vi "0816039.vi"() -> ()   [LabVIEW 2021]
panel:
  out "M2":string
  out "M1":string
  out "elapsed\ntime":u32
  out "current time":timestamp format="%<%X %x>T"
  in  "stop":bool
  out "Display":string
  in  "Calculator":T1
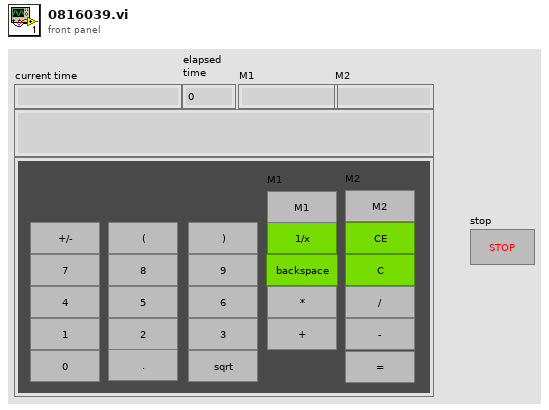
[diagram p1: front panel]
types:
  T1 = cluster{"1":bool, "2":bool, "3":bool, "4":bool, "5":bool, "6":bool, "7":bool, "8":bool, "9":bool, "+":bool, "-":bool, "*":bool, "/":bool, "C":bool, "=":bool, "0":bool, ".":bool, "(":bool, ")":bool, "backspace":bool, "1/x":bool, "CE":bool, "sqrt":bool, "+/-":bool, "M1":bool, "M2":bool}
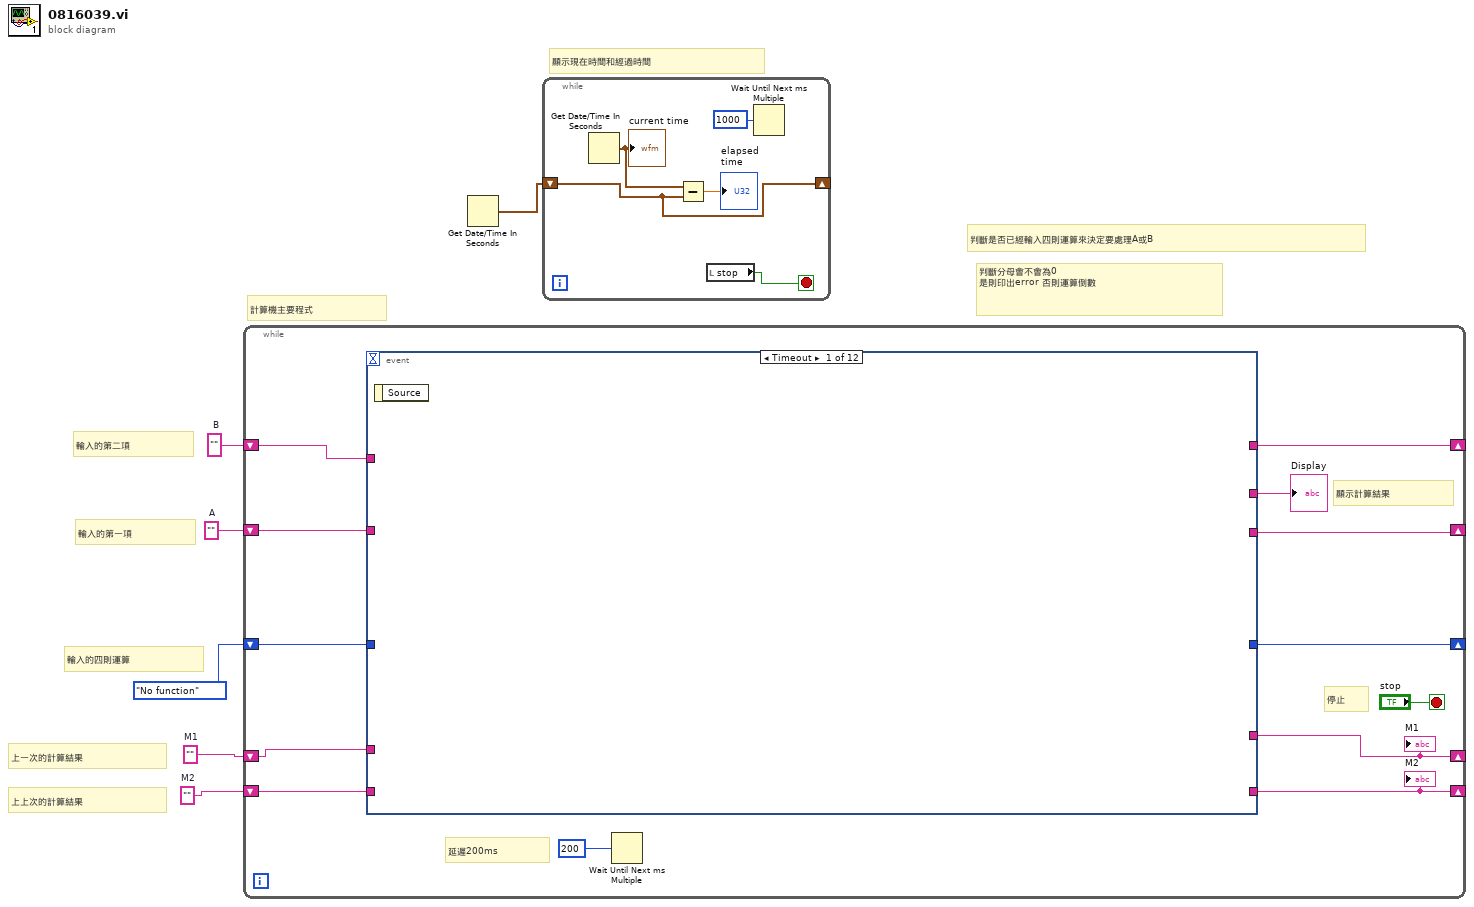
[diagram p0: block diagram]
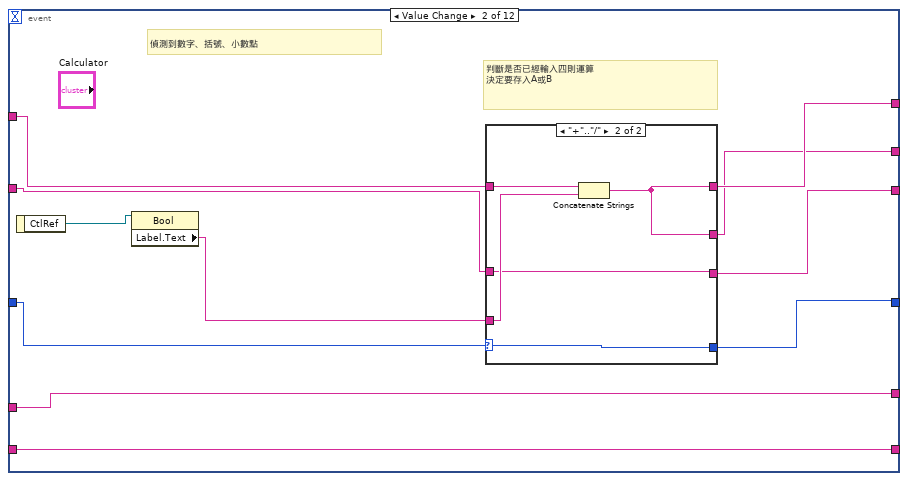
[diagram p2: hidden frame]
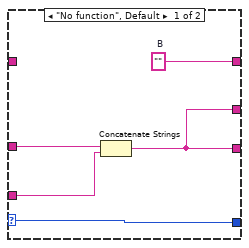
[diagram p3: hidden frame]
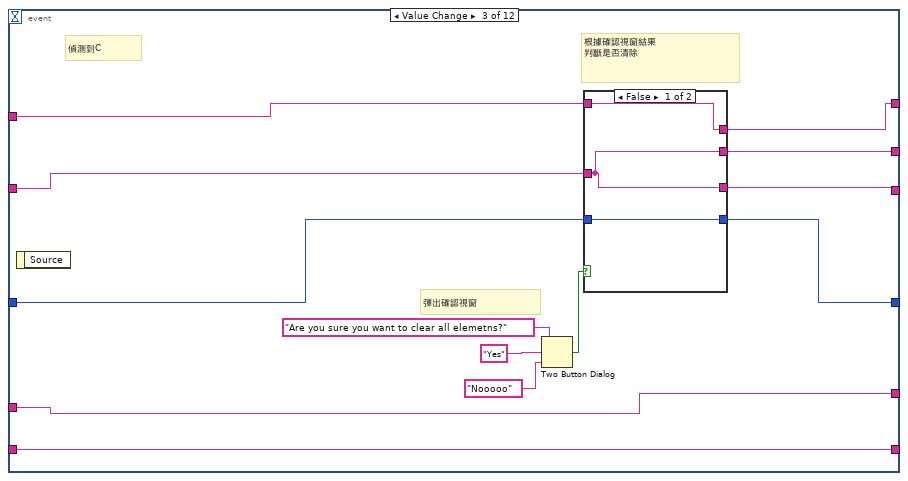
[diagram p4: hidden frame]
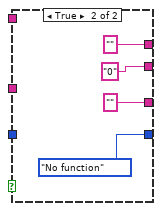
[diagram p5: hidden frame]
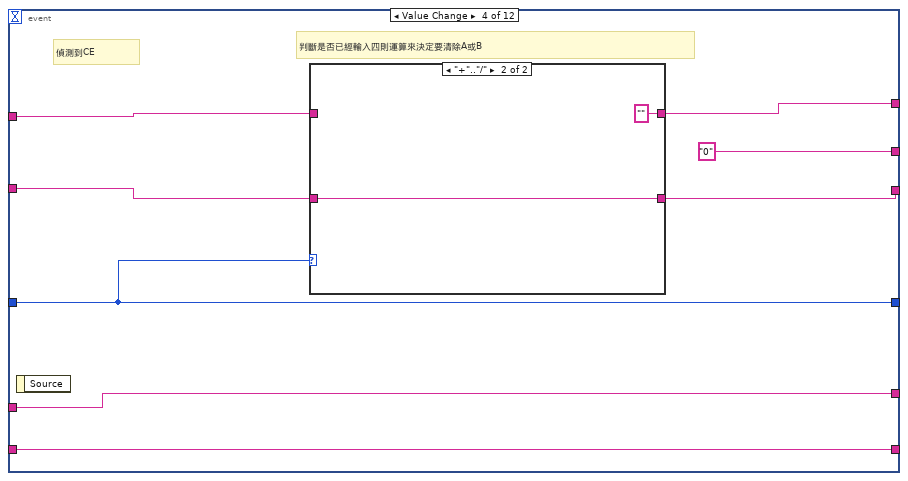
[diagram p6: hidden frame]
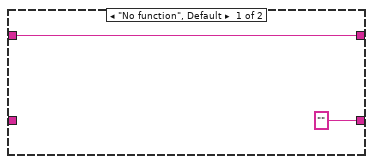
[diagram p7: hidden frame]
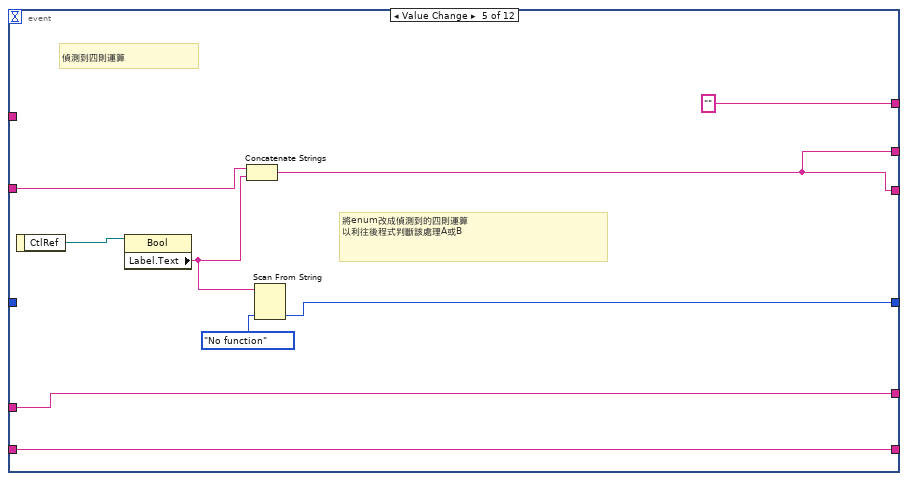
[diagram p8: hidden frame]
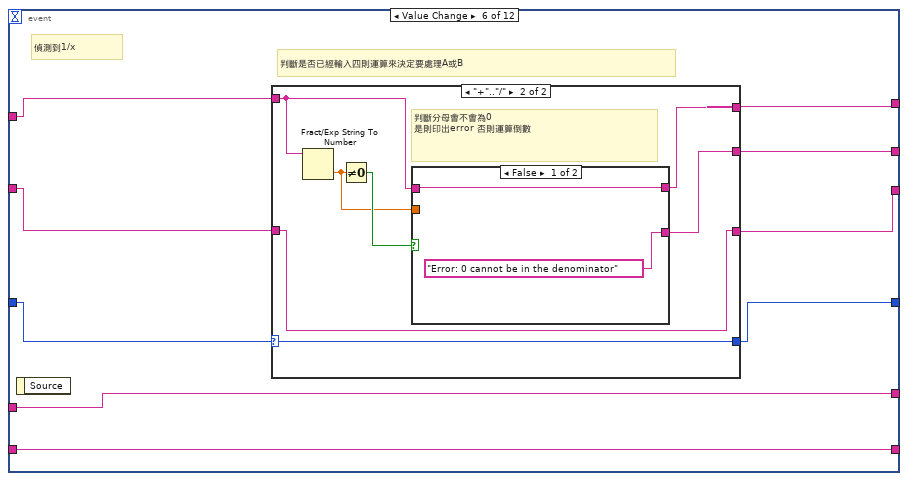
[diagram p9: hidden frame]
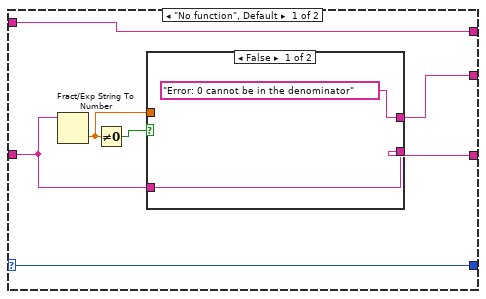
[diagram p10: hidden frame]
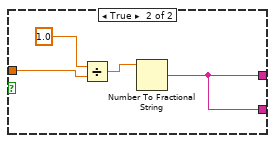
[diagram p11: hidden frame]
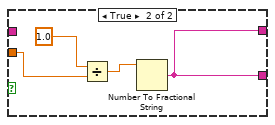
[diagram p12: hidden frame]
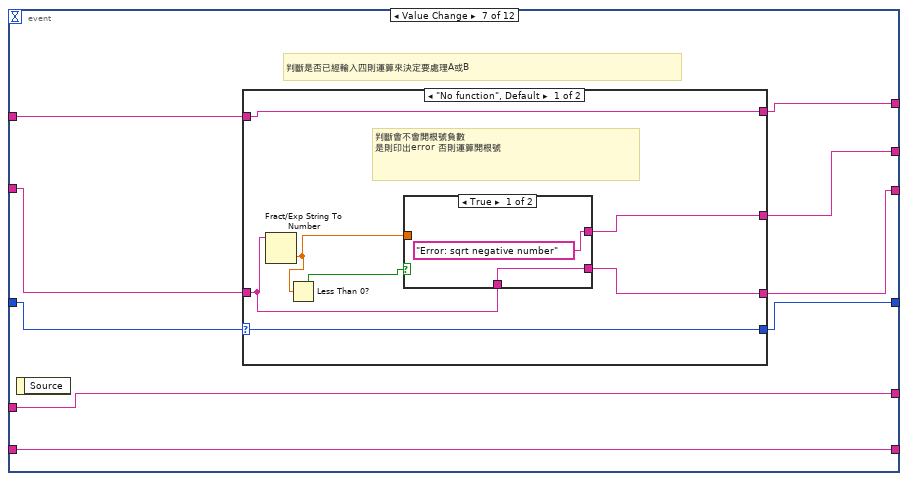
[diagram p13: hidden frame]
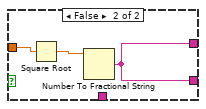
[diagram p14: hidden frame]
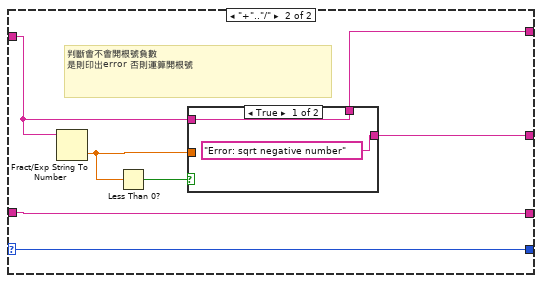
[diagram p15: hidden frame]
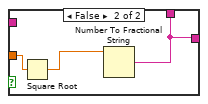
[diagram p16: hidden frame]
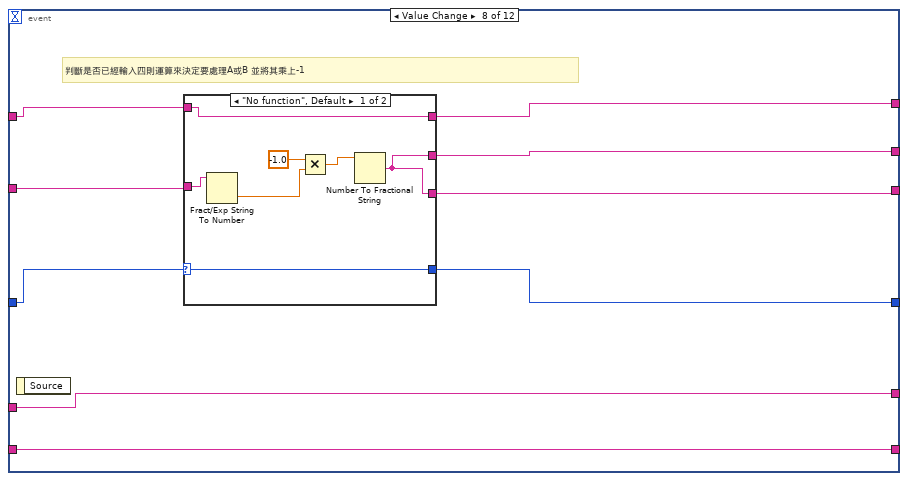
[diagram p17: hidden frame]
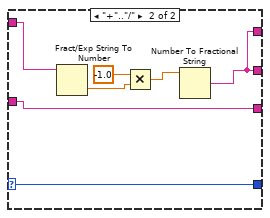
[diagram p18: hidden frame]
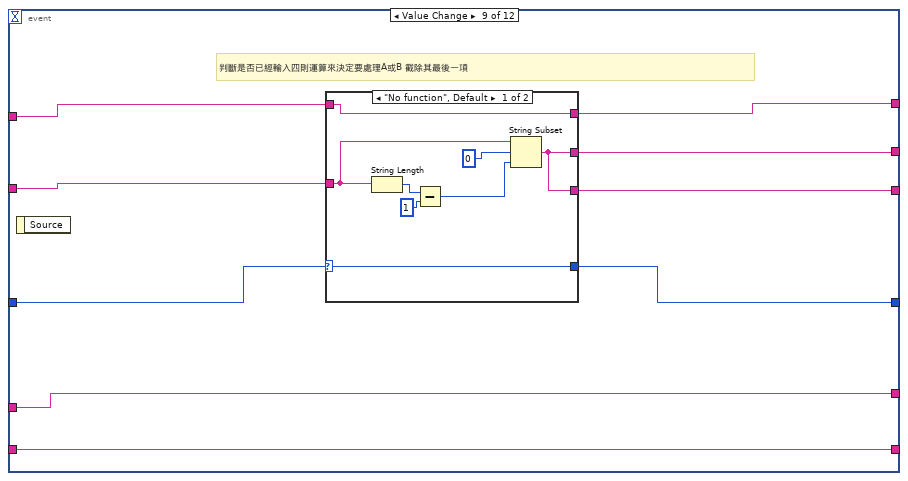
[diagram p19: hidden frame]
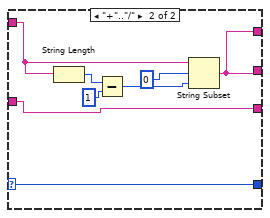
[diagram p20: hidden frame]
diagram:
  w1 = ""  # M2
  w2 = ""  # M1
  w5 = ""  # A
  w6 = ""  # B
  # "判斷是否已經輸入四則運算來決定要處理A或B"
  # "判斷分母會不會為0\n是則印出error 否則運算倒數"
  # "上上次的計算結果"
  # "上一次的計算結果"
  # "輸入的四則運算"
  # "輸入的第二項"
  # "輸入的第一項"
  # "計算機主要程式"
  # "顯示現在時間和經過時間"
  n1 = while {
    shift-right: [w15] -> _
    shift-left: w6 -> [w19]
    shift-right: [w16] -> _
    shift-left: w5 -> [w18]
    shift-right: [w14] -> _
    shift-left: enum16{"No function", "+", "-", "*", "/", "C"}."No function" -> [w17]
    shift-right: [w8] -> _
    shift-left: w2 -> [w12]
    shift-right: [w11] -> _
    shift-left: w1 -> [w9]
    stop <- "stop" stop-if-true
    # "停止"
    # "顯示計算結果"
    # "延遲200ms"
    n2 = event shown="[0] Timeout" {
      selector: _ -> [_ _ _ _ _ _ _ _ _ _ _ _]
      dyn-events: _ -> [_ _ _ _ _ _ _ _ _ _ _ _]
      timeout: _ -> [_ _ _ _ _ _ _ _ _ _ _ _]
      tunnel: w19 -> [_ w21 w45 w65 _ w90 w125 w158 w177 w204 _ _]
      tunnel: w18 -> [_ w20 w44 w63 w77 w89 w124 w157 w180 w203 _ _]
      tunnel: w17 -> [_ w25 w43 w61 _ w88 w118 w156 w181 w205 _ _]
      tunnel: [_ w24 w46 w61 w80 w85 w117 w153 w175 enum16{"No function", "+", "-", "*", "/", "C"}."No function" _ _] -> w14
      tunnel: [_ w28 w47 w62 w76 w86 w122 w154 w178 w200 _ _] -> w16
      tunnel: [_ w27 w49 w64 "" ("B") w87 w123 w155 w176 w201 _ _] -> w15
      tunnel: [_ w26 w48 "0" ("B") w76 w84 w121 w152 w179 w198 w246 w247] -> w10
      tunnel: w12 -> [_ w23 w42 w67 w74 w83 w120 w151 w174 w199 w246 w248]
      tunnel: [_ w22 w41 w66 w73 w82 w119 w150 w173 w199 w245 w247] -> w11
      tunnel: w9 -> [_ w22 w41 w66 w73 w82 w119 w150 w173 _ w245 w247]
      tunnel: [_ w23 w42 w67 w74 w83 w120 w151 w174 w198 w246 w248] -> w8
      event Timeout {
        n3 = event-data() -> ()  [unwired: 1 in, 1 out]
      }
      event "Calculator.0", "Calculator.1", "Calculator.2", "Calculator.3", "Calculator.4", "Calculator.5", "Calculator.6", "Calculator.7", "Calculator.8", "Calculator.9", "Calculator..", "Calculator.(", "Calculator.)": Value Change {
        # "判斷是否已經輸入四則運算\n決定要存入A或B"
        # "偵測到數字、括號、小數點"
        n4 = event-data() -> ("CtlRef"=w30:refnum<vi>)  [unwired: 1 in]
        n5 = property class="Bool"(reference=w30) -> ("Label.Text"=w29:string)  [unwired: 1 in, 2 out]
        n6 = case shown="\"+\"..\"/\"" w25 {
          selector: w25 -> [w31 w36]
          tunnel: w20 -> [w35 w38]
          tunnel: w29 -> [w34 w39]
          tunnel: [w32 w38] -> w28
          tunnel: w21 -> [_ w40]
          tunnel: [w33 w37] -> w27
          tunnel: [w32 w37] -> w26
          tunnel: [w31 w36] -> w24
          frame "No function", Default {
            w33 = ""  # B
            n7 = Concatenate Strings(w35, w34) -> (w32:string)
          }
          frame "+".."/" {
            n8 = Concatenate Strings(w40, w39) -> (w37:string)
          }
        }
      }
      event "Calculator.C": Value Change {
        # "根據確認視窗結果\n判斷是否清除"
        # "彈出確認視窗"
        # "偵測到C"
        n9 = event-data() -> ()  [unwired: 1 in, 1 out]
        n10 = Two Button Dialog(message="Are you sure you want to clear all elemetns?" ("F button name (\"Cancel\")"), 1:"Nooooo" ("F button name (\"Cancel\")"), 2:"Yes" ("T button name (\"OK\")")) -> (T button?=w50:bool)
        n11 = case shown="False" w50 {
          tunnel: [w56 "" ("B")] -> w49
          tunnel: [w55 "0" ("B")] -> w48
          tunnel: [w55 "" ("A")] -> w47
          tunnel: [w54 enum16{"No function", "+", "-", "*", "/", "C"}."No function"] -> w46
          tunnel: w45 -> [w56 _]
          tunnel: w44 -> [w55 _]
          tunnel: w43 -> [w54 _]
          frame False {
          }
          frame True {
          }
        }
      }
      event "Calculator.CE": Value Change {
        # "判斷是否已經輸入四則運算來決定要清除A或B"
        # "偵測到CE"
        n12 = event-data() -> ()  [unwired: 1 in, 1 out]
        n13 = case shown="\"+\"..\"/\"" w61 {
          tunnel: [w70 "" ("B")] -> w64
          tunnel: w65 -> [w70 _]
          tunnel: w63 -> [_ w72]
          tunnel: ["" w72] -> w62
          frame "No function", Default {
          }
          frame "+".."/" {
          }
        }
      }
      event "Calculator.+", "Calculator.-", "Calculator.*", "Calculator./": Value Change {
        # "將enum改成偵測到的四則運算\n以利往後程式判斷該處理A或B"
        # "偵測到四則運算"
        n14 = event-data() -> ("CtlRef"=w81:refnum<vi>)  [unwired: 1 in]
        n15 = property class="Bool"(reference=w81) -> ("Label.Text"=w75:string)  [unwired: 1 in, 2 out]
        n16 = Concatenate Strings(w77, w75) -> (w76:string)
        n17 = Scan From String(input string=w75, default 1=enum16{"No function", "+", "-", "*", "/"}."No function") -> (output 1=w80:enum16{"No function", "+", "-", "*", "/"})  [unwired: 3 in, 3 out]
      }
      event "Calculator.1/x": Value Change {
        # "判斷是否已經輸入四則運算來決定要處理A或B"
        # "偵測到1/x"
        n18 = event-data() -> ()  [unwired: 1 in, 1 out]
        n19 = case shown="\"+\"..\"/\"" w88 {
          selector: w88 -> [w96 w110]
          tunnel: w89 -> [w91 w105]
          tunnel: [w92 w105] -> w86
          tunnel: w90 -> [w97 w106]
          tunnel: [w97 w104] -> w87
          tunnel: [w96 w110] -> w85
          tunnel: [w93 w107] -> w84
          frame "No function", Default {
            n20 = Fract/Exp String To Number(string=w91) -> (number=w94:dbl)  [unwired: 3 in, 1 out]
            n21 = Not Equal To 0?(x=w94) -> (x != 0?=w95:bool)
            n22 = case shown="False" w95 {
              tunnel: w94 -> [_ w101]
              tunnel: ["Error: 0 cannot be in the denominator" w100] -> w93
              tunnel: [w99 w100] -> w92
              tunnel: w91 -> [w99 _]
              frame False {
              }
              frame True {
                n23 = Divide(x=1.0 ("y"), y=w101) -> (x/y=w102:dbl)
                n24 = Number To Fractional String(number=w102) -> (F-format string=w100:string)  [unwired: 3 in]
              }
            }
          }
          frame "+".."/" {
            # "判斷分母會不會為0\n是則印出error 否則運算倒數"
            n25 = Fract/Exp String To Number(string=w106) -> (number=w108:dbl)  [unwired: 3 in, 1 out]
            n26 = Not Equal To 0?(x=w108) -> (x != 0?=w109:bool)
            n27 = case shown="False" w109 {
              tunnel: w108 -> [_ w114]
              tunnel: ["Error: 0 cannot be in the denominator" w113] -> w107
              tunnel: [w111 w113] -> w104
              tunnel: w106 -> [w111 _]
              frame False {
              }
              frame True {
                n28 = Divide(x=1.0 ("y"), y=w114) -> (x/y=w115:dbl)
                n29 = Number To Fractional String(number=w115) -> (F-format string=w113:string)  [unwired: 3 in]
              }
            }
          }
        }
      }
      event "Calculator.sqrt": Value Change {
        # "判斷是否已經輸入四則運算來決定要處理A或B"
        n30 = event-data() -> ()  [unwired: 1 in, 1 out]
        n31 = case shown="\"No function\", Default" w118 {
          selector: w118 -> [w131 w144]
          tunnel: w124 -> [w126 w143]
          tunnel: [w127 w143] -> w122
          tunnel: w125 -> [w132 w138]
          tunnel: [w132 w139] -> w123
          tunnel: [w131 w144] -> w117
          tunnel: [w128 w140] -> w121
          frame "No function", Default {
            # "判斷會不會開根號負數\n是則印出error 否則運算開根號"
            n32 = Fract/Exp String To Number(string=w126) -> (number=w129:dbl)  [unwired: 3 in, 1 out]
            n33 = Less Than 0?(x=w129) -> (x < 0?=w130:bool)
            n34 = case shown="True" w130 {
              tunnel: w129 -> [_ w137]
              tunnel: ["Error: sqrt negative number" w135] -> w128
              tunnel: [w133 w135] -> w127
              tunnel: w126 -> [w133 _]
              frame True {
              }
              frame False {
                n35 = Square Root(x=w137) -> (sqrt(x)=w136:dbl)
                n36 = Number To Fractional String(number=w136) -> (F-format string=w135:string)  [unwired: 3 in]
              }
            }
          }
          frame "+".."/" {
            # "判斷會不會開根號負數\n是則印出error 否則運算開根號"
            n37 = Fract/Exp String To Number(string=w138) -> (number=w142:dbl)  [unwired: 3 in, 1 out]
            n38 = Less Than 0?(x=w142) -> (x < 0?=w141:bool)
            n39 = case shown="True" w141 {
              tunnel: w142 -> [_ w149]
              tunnel: ["Error: sqrt negative number" w147] -> w140
              tunnel: [w145 w147] -> w139
              tunnel: w138 -> [w145 _]
              frame True {
              }
              frame False {
                n40 = Square Root(x=w149) -> (sqrt(x)=w148:dbl)
                n41 = Number To Fractional String(number=w148) -> (F-format string=w147:string)  [unwired: 3 in]
              }
            }
          }
        }
      }
      event "Calculator.+/-": Value Change {
        # "判斷是否已經輸入四則運算來決定要處理A或B 並將其乘上-1"
        n42 = event-data() -> ()  [unwired: 1 in, 1 out]
        n43 = case shown="\"No function\", Default" w156 {
          selector: w156 -> [w164 w172]
          tunnel: w157 -> [w163 w168]
          tunnel: [w160 w168] -> w154
          tunnel: w158 -> [w165 w169]
          tunnel: [w165 w167] -> w155
          tunnel: [w164 w172] -> w153
          tunnel: [w160 w167] -> w152
          frame "No function", Default {
            n44 = Fract/Exp String To Number(string=w163) -> (number=w162:dbl)  [unwired: 3 in, 1 out]
            n45 = Multiply(x=-1.0, y=w162) -> (x*y=w161:dbl)
            n46 = Number To Fractional String(number=w161) -> (F-format string=w160:string)  [unwired: 3 in]
          }
          frame "+".."/" {
            n47 = Fract/Exp String To Number(string=w169) -> (number=w171:dbl)  [unwired: 3 in, 1 out]
            n48 = Multiply(x=-1.0, y=w171) -> (x*y=w170:dbl)
            n49 = Number To Fractional String(number=w170) -> (F-format string=w167:string)  [unwired: 3 in]
          }
        }
      }
      event "Calculator.backspace": Value Change {
        # "判斷是否已經輸入四則運算來決定要處理A或B 截除其最後一項"
        n50 = event-data() -> ()  [unwired: 1 in, 1 out]
        n51 = case shown="\"No function\", Default" w181 {
          selector: w181 -> [w182 w190]
          tunnel: w180 -> [w184 w191]
          tunnel: [w185 w193] -> w179
          tunnel: [w185 w191] -> w178
          tunnel: w177 -> [w183 w192]
          tunnel: [w183 w193] -> w176
          tunnel: [w182 w190] -> w175
          frame "No function", Default {
            n52 = String Length(string=w184) -> (length=w188:i32)
            n53 = Subtract(x=w188, y=1 ("x-y")) -> (x-y=w186:i32)
            n54 = String Subset(string=w184, offset (0)=0, length (rest)=w186) -> (substring=w185:string)
          }
          frame "+".."/" {
            n55 = String Length(string=w192) -> (length=w196:i32)
            n56 = Subtract(x=w196, y=1 ("x-y")) -> (x-y=w194:i32)
            n57 = String Subset(string=w192, offset (0)=0, length (rest)=w194) -> (substring=w193:string)
          }
        }
      }
      event "Calculator.=": Value Change {
        # "判斷輸入的四則運算"
        n58 = event-data() -> ()  [unwired: 1 in, 1 out]
        n59 = case shown="\"/\"" w205 {
          tunnel: w204 -> [w207 w215 w221 w227 w238]
          tunnel: w203 -> [w206 w214 w222 w228 w239]
          tunnel: [w206 w210 w220 w226 w237] -> w198
          tunnel: [w207 "" "" "" ""] -> w201
          tunnel: [w206 "" "" "" ""] -> w200
          frame Default {
            # "未輸入四則運算 保留輸入的第一項"
          }
          frame "+" {
            # "執行加法＆清除輸入項"
            n60 = Fract/Exp String To Number(string=w214) -> (number=w212:dbl)  [unwired: 3 in, 1 out]
            n61 = Fract/Exp String To Number(string=w215) -> (number=w213:dbl)  [unwired: 3 in, 1 out]
            n62 = Add(x=w213, y=w212) -> (x+y=w211:dbl)
            n63 = Number To Fractional String(number=w211) -> (F-format string=w210:string)  [unwired: 3 in]
          }
          frame "-" {
            # "執行減法＆清除輸入項"
            n64 = Fract/Exp String To Number(string=w222) -> (number=w219:dbl)  [unwired: 3 in, 1 out]
            n65 = Fract/Exp String To Number(string=w221) -> (number=w216:dbl)  [unwired: 3 in, 1 out]
            n66 = Subtract(x=w219, y=w216) -> (x-y=w223:dbl)
            n67 = Number To Fractional String(number=w223) -> (F-format string=w220:string)  [unwired: 3 in]
          }
          frame "*" {
            # "執行乘法＆清除輸入項"
            n68 = Fract/Exp String To Number(string=w228) -> (number=w230:dbl)  [unwired: 3 in, 1 out]
            n69 = Fract/Exp String To Number(string=w227) -> (number=w231:dbl)  [unwired: 3 in, 1 out]
            n70 = Multiply(x=w231, y=w230) -> (x*y=w229:dbl)
            n71 = Number To Fractional String(number=w229) -> (F-format string=w226:string)  [unwired: 3 in]
          }
          frame "/" {
            # "判斷除數會不會為0\n是則印出error 否則運算除法"
            # "執行除法＆清除輸入項"
            n72 = Fract/Exp String To Number(string=w238) -> (number=w233:dbl)  [unwired: 3 in, 1 out]
            n73 = Fract/Exp String To Number(string=w239) -> (number=w236:dbl)  [unwired: 3 in, 1 out]
            n74 = Equal To 0?(x=w233) -> (x = 0?=w232:bool)
            n75 = case shown="True" w232 {
              tunnel: ["Error: divided by zero" w243] -> w237
              tunnel: w236 -> [_ w242]
              tunnel: w233 -> [_ w241]
              frame True {
              }
              frame False {
                n76 = Divide(x=w242, y=w241) -> (x/y=w244:dbl)
                n77 = Number To Fractional String(number=w244) -> (F-format string=w243:string)  [unwired: 3 in]
              }
            }
          }
        }
      }
      event "Calculator.M1": Value Change {
        # "顯示上次的計算結果"
        n78 = event-data() -> ()  [unwired: 1 in, 1 out]
      }
      event "Calculator.M2": Value Change {
        # "顯示上上次的計算結果"
        n79 = event-data() -> ()  [unwired: 1 in, 1 out]
      }
    }
    "Display" <- w10
    "M1" <- w8
    "M2" <- w11
    n80 = Wait Until Next ms Multiple(millisecond multiple=u32 200) -> ()  [unwired: 1 out]
  }
  n81 = Get Date/Time In Seconds() -> (seconds since 1Jan1904=w3:timestamp)
  n82 = while {
    shift-right: [w249] -> _
    shift-left: w3 -> [w249]
    stop <- w253 stop-if-true
    n83 = Get Date/Time In Seconds() -> (seconds since 1Jan1904=w251:timestamp)
    "current time" <- w251
    n84 = Subtract(x=w251, y=w249) -> (x-y=→"elapsed\ntime":dbl)
    n85 = local read "stop"() -> (w253:bool)
    n86 = Wait Until Next ms Multiple(millisecond multiple=1000) -> ()  [unwired: 1 out]
  }
